vi "connection counter.vi"() -> (3 "id":i32)   [LabVIEW 2016, in "websocket upgrade handler.lvclass"]
uses:
  websocket upgrade handler.lvclass
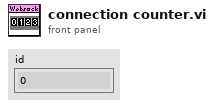
[diagram p1: front panel]
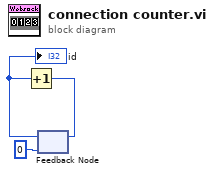
[diagram p0: block diagram]
diagram:
  n1 = feedback #1(0) -> (w2:i32)
  "id" <- w2
  n2 = Increment(x=w2) -> (x+1=w1:i32)
  n3 = feedback-in #1(w1) -> ()
